vi "Select.vi"(10 "Tabla":string="Tabla1") -> (2 "String":string)   [LabVIEW 2012]
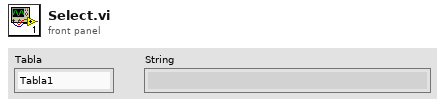
[diagram p1: front panel]
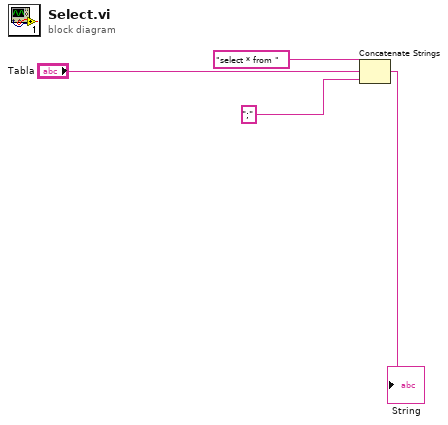
[diagram p0: block diagram]
diagram:
  n1 = Concatenate Strings("select * from " ("SQL query"), "Tabla", ";" ("Substring")) -> (→"String":string)
